vi "Global.vi"() -> ()   [LabVIEW 2016]
uses:
  SensorInfo.ctl
panel:
  out "显示坐标信息":T1
  in  "温湿度数值":string[][](table)
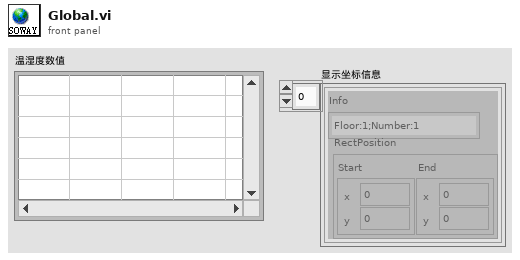
[diagram p1: front panel]
types:
  T1 = typedef "SensorInfo.ctl" = cluster{"Info":string, "RectPosition":cluster{"Start":cluster{"x":i16, "y":i16}, "End":cluster{"x":i16, "y":i16}}}[]
diagram:
